vi "Check If Has ExcuseNote.vi"(6 "Determine(\"\")":string, 7 "Time(\"\")":string, 8 "error in (no error)":errorcluster, 9 "ExcuseNote(\"\")":string, 10 "Date":string, 11 "List":string[][](array[string])) -> (0 "error out":errorcluster, 3 "2D Array":string[][](array[string]))   [LabVIEW 2015, in "Admin_Actor.lvlib" / "ExcuseNotesHandler.lvclass"]
uses:
  ExcuseNotesHandler.lvclass
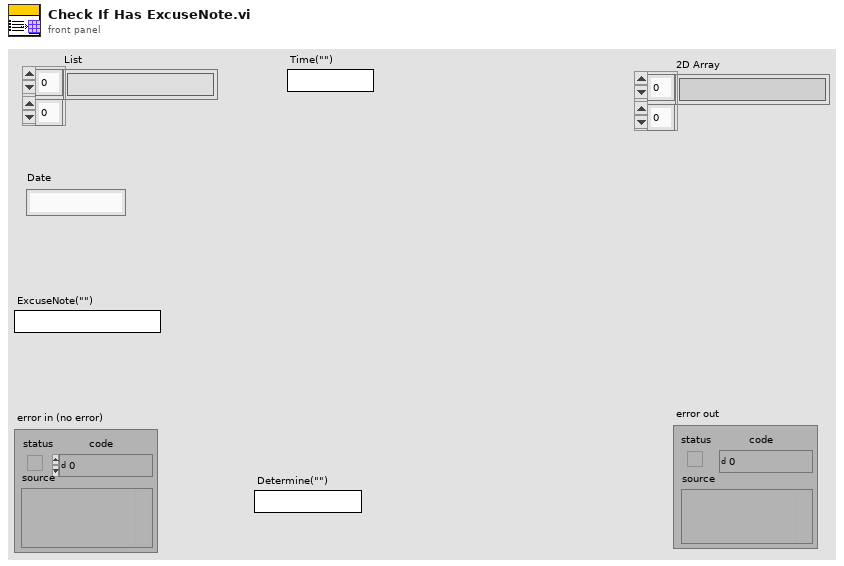
[diagram p1: front panel]
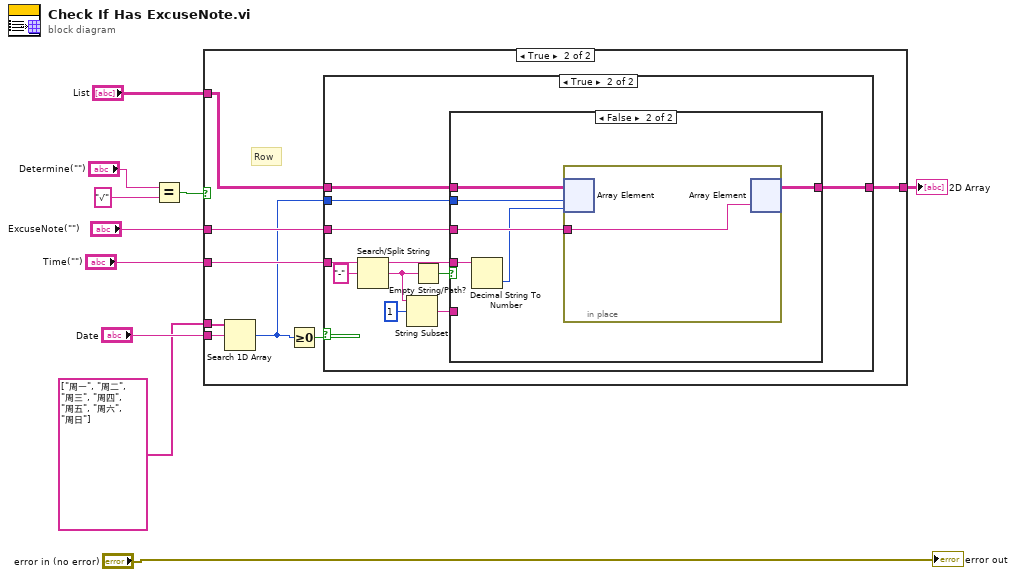
[diagram p0: block diagram]
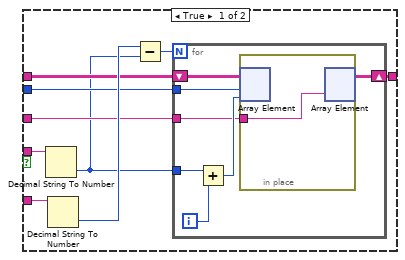
[diagram p4: hidden frame]
diagram:
  n1 = Equal?(x="Determine(\"\")", y="√") -> (x = y?=w8:bool)
  n2 = case shown="True" w8 {
    tunnel: "Time(\"\")" -> [_ w15]
    tunnel: "List" -> [w11 w19]
    tunnel: "Date" -> [_ w18]
    tunnel: string[] ["周一", "周二", "周三", "周四", "周五", "周六", "周日"] -> [_ w17]
    tunnel: "ExcuseNote(\"\")" -> [_ w14]
    tunnel: [w11 w12] -> w2
    frame False {
    }
    frame True {
      # "Row"
      n3 = Search 1D Array(1D array=w17, element=w18) -> (index of element=w13:i32)  [unwired: 1 in]
      n4 = Greater Or Equal To 0?(x=w13) -> (x >= 0?=w16:bool)
      n5 = case shown="True" w16 {
        tunnel: w19 -> [w20 w24]
        tunnel: w15 -> [_ w31]
        tunnel: w14 -> [_ w25]
        tunnel: w13 -> [_ w23]
        tunnel: [w20 w22] -> w12
        frame False {
        }
        frame True {
          n6 = Search/Split String(string=w31, search string/char (-)="-") -> (substring before match=w29:string, match + rest of string=w28:string)  [unwired: 1 in, 1 out]
          n7 = String Subset(string=w28, offset (0)=1) -> (substring=w26:string)  [unwired: 1 in]
          n8 = Empty String/Path?(string/path=w28) -> (empty?=w30:bool)
          n9 = case shown="False" w30 {
            tunnel: w29 -> [w40 w54]
            tunnel: w26 -> [w39 _]
            tunnel: w24 -> [w36 w53]
            tunnel: w25 -> [w35 w52]
            tunnel: w23 -> [w34 w51]
            tunnel: [w32 w49] -> w22
            frame True {
              n10 = Decimal String To Number(string=w40) -> (number=w33:i32)  [unwired: 2 in, 1 out]
              n11 = Decimal String To Number(string=w39) -> (number=w38:i32)  [unwired: 2 in, 1 out]
              n12 = Subtract(x=w38, y=w33) -> (x-y=w37:i32)
              n13 = for {
                N: w37 -> [_]
                tunnel: w35 -> [w42]
                tunnel: w34 -> [w46]
                tunnel: w33 -> [w45]
                shift-right: [w41] -> w32
                shift-left: w36 -> [w47]
                i -> [w44]
                n14 = Add(x=w45, y=w44) -> (x+y=w43:i32)
                n15 = in-place {
                  in-place-border: w42 -> [w48]
                  n16 = in-place-array #1(w47, w46, w43) -> ()  [unwired: 1 out]
                  n17 = in-place-array #1(w48) -> (w41:string[][])  [unwired: 2 out]
                }
              }
            }
            frame False {
              n18 = Decimal String To Number(string=w54) -> (number=w50:i32)  [unwired: 2 in, 1 out]
              n19 = in-place {
                in-place-border: w52 -> [w55]
                n20 = in-place-array #2(w53, w51, w50) -> ()  [unwired: 1 out]
                n21 = in-place-array #2(w55) -> (w49:string[][])  [unwired: 2 out]
              }
            }
          }
        }
      }
    }
  }
  "2D Array" <- w2
  "error out" <- "error in (no error)"
